vi "subSetExternalLibDependencies.vi"(8 "error in (no error)":errorcluster, 11 "SolutionBuilder in":refnum<class "SolutionBuilder.lvclass">) -> (0 "error out":errorcluster, 3 "SolutionBuilder out":refnum<class "SolutionBuilder.lvclass">)   [LabVIEW 2019, in "SolutionBuilder.lvlib" / "SolutionBuilder.lvclass"]
uses:
  SolutionBuilder.lvclass
  SolutionBuilder.lvclass/SolutionBuilder.ctl
  ProjectItem/ProjectItem.lvclass
  <vilib>/Utility/LVLibp/NI_PackedLibraryUtility.lvlib
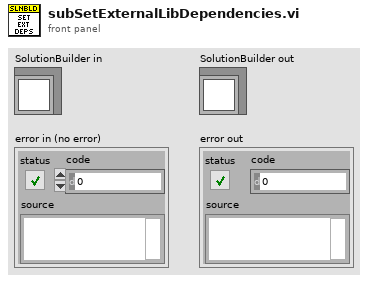
[diagram p1: front panel]
types:
  T1 = typedef "SolutionBuilder.lvlib/SolutionBuilder.lvclass/ProjectItemMap.ctl" = map{path, refnum<class "ProjectItem.lvclass">[]}
  T2 = typedef "SolutionBuilder.lvlib/SolutionBuilder.lvclass/NamePathMap.ctl" = map{string, path}
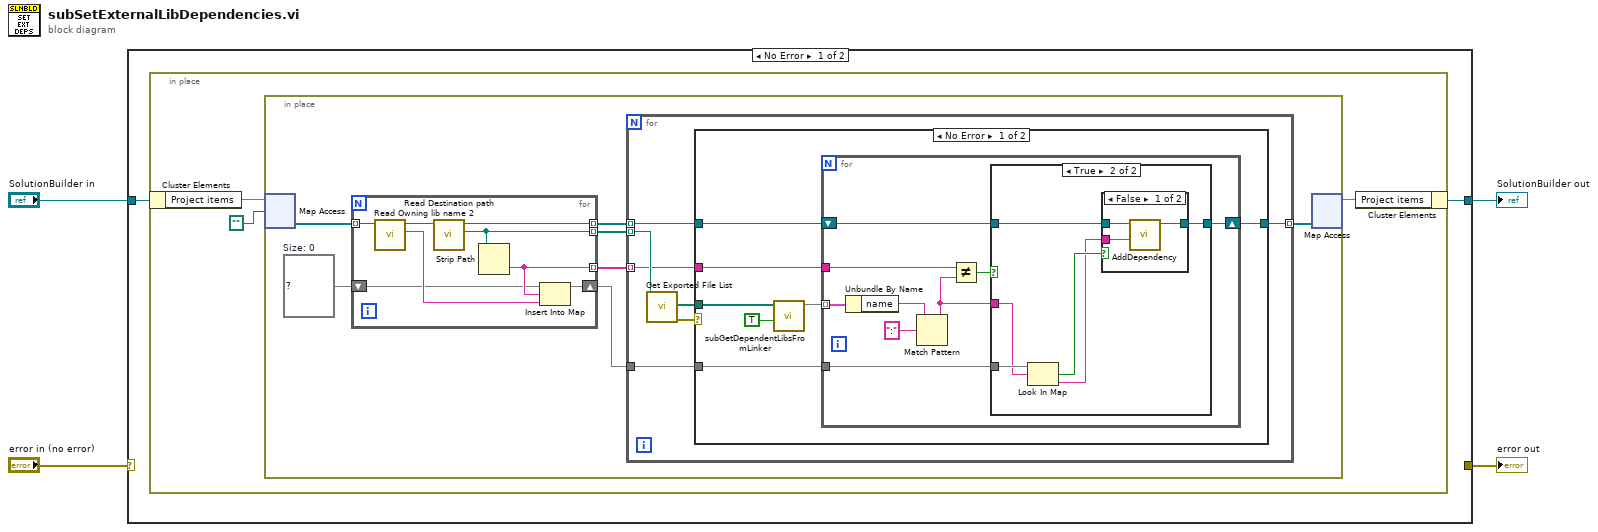
[diagram p0: block diagram]
diagram:
  n1 = case shown="No Error" "error in (no error)" {
    selector: "error in (no error)" -> [_ w61]
    tunnel: [_ w61] -> w3
    tunnel: [w6 w60] -> w2
    tunnel: "SolutionBuilder in" -> [w5 w60]
    frame No Error {
      n2 = in-place {
        n3 = in-place-cluster #1(w5) -> ("Project items"=w9:T1)
        n4 = in-place {
          w11 = map{string, string} {}  # Size: 0
          n5 = in-place-map #2(w9, path "") -> (w15:refnum<class "ProjectItem.lvclass">[])  [unwired: 1 in, 1 out]
          n6 = for {
            tunnel: w15 -> [w22] mode=indexing
            tunnel: [w24] -> w14 mode=indexing
            tunnel: [w20] -> w12 mode=indexing
            tunnel: [w23] -> w13 mode=indexing
            shift-right: [w18] -> w10
            shift-left: w11 -> [w17]
            n7 = call "Read Owning lib name 2.vi"("ProjectItem in"=w22) -> ("Owning lib name"=w19:string, "ProjectItem out"=w21:refnum<class "ProjectItem.lvclass">)  [unwired: 9 in]
            n8 = call "Read Destination path.vi"("ProjectItem in"=w21) -> ("Destination path"=w23:path, "ProjectItem out"=w24:refnum<class "ProjectItem.lvclass">)  [unwired: 9 in]
            n9 = Strip Path(path=w23) -> (name=w20:string)  [unwired: 1 out]
            n10 = Insert Into Map(map in=w17, key=w20, value=w19) -> (map out=w18:map{string, string})  [unwired: 2 out]
          }
          n11 = for {
            tunnel: w14 -> [w28] mode=indexing
            tunnel: [w29] -> w16 mode=indexing
            tunnel: w13 -> [w27] mode=indexing
            tunnel: w12 -> [w26] mode=indexing
            tunnel: w10 -> [w25]
            n12 = call <vilib>:"Get Exported File List.vi"("packed library path"=w27) -> ("error out"=w31:errorcluster, "paths"=w30:path[])  [unwired: 8 in, 1 out]
            n13 = case shown="No Error" w31 {
              tunnel: w30 -> [w37 _]
              tunnel: w28 -> [w34 w59]
              tunnel: [w36 w59] -> w29
              tunnel: w26 -> [w33 _]
              tunnel: w25 -> [w32 _]
              frame No Error {
                n14 = call "subGetDependentLibsFromLinker.vi"("All?"=TRUE, "Paths"=w37) -> ("Dependency libs"=w35:T2)  [unwired: 8 in, 1 out]
                n15 = for {
                  tunnel: w35 -> [w45] mode=indexing
                  shift-right: [w46] -> w36
                  shift-left: w34 -> [w47]
                  tunnel: w33 -> [w42]
                  tunnel: w32 -> [w39]
                  n16 = Unbundle By Name(w45) -> ("name"=w44:string)
                  n17 = Match Pattern(string=w44, regular expression=":") -> (before substring=w41:string)  [unwired: 1 in, 3 out]
                  n18 = Not Equal?(x=w42, y=w41) -> (x != y?=w40:bool)
                  n19 = case shown="True" w40 {
                    tunnel: w47 -> [w48 w54]
                    tunnel: [w48 w53] -> w46
                    tunnel: w41 -> [_ w51]
                    tunnel: w39 -> [_ w52]
                    frame False {
                    }
                    frame True {
                      n20 = Look In Map(map=w52, key=w51) -> (key not found?=w50:bool, value=w49:string)  [unwired: 1 in]
                      n21 = case shown="False" w50 {
                        tunnel: w54 -> [w57 w58]
                        tunnel: [w56 w58] -> w53
                        tunnel: w49 -> [w55 _]
                        frame False {
                          n22 = call "AddDependency.vi"("Dependency"=w55, "ProjectItem in"=w57) -> ("ProjectItem out"=w56:refnum<class "ProjectItem.lvclass">)  [unwired: 8 in, 1 out]
                        }
                        frame True {
                        }
                      }
                    }
                  }
                }
              }
              frame Error {
              }
            }
          }
          n23 = in-place-map #2(w16) -> (w7:T1)  [unwired: 1 in, 2 out]
        }
        n24 = in-place-cluster #1("Project items"=w7) -> (w6:refnum<class "SolutionBuilder.lvclass">)
      }
    }
    frame Error {
    }
  }
  "error out" <- w3
  "SolutionBuilder out" <- w2
